vi "Dequeue if val.vi"(8 "error in (no error)":errorcluster, 11 "Queue in":refnum<queue>) -> (0 "error out":errorcluster, 3 "Queue out":refnum<queue>, 4 "Marin Serial Response":string)   [LabVIEW 2020]
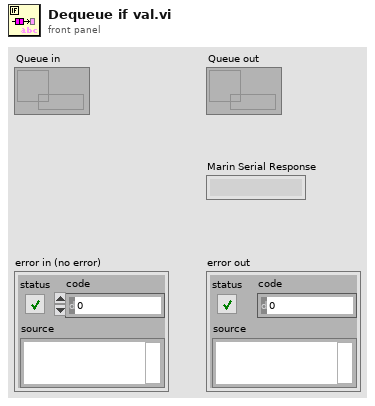
[diagram p1: front panel]
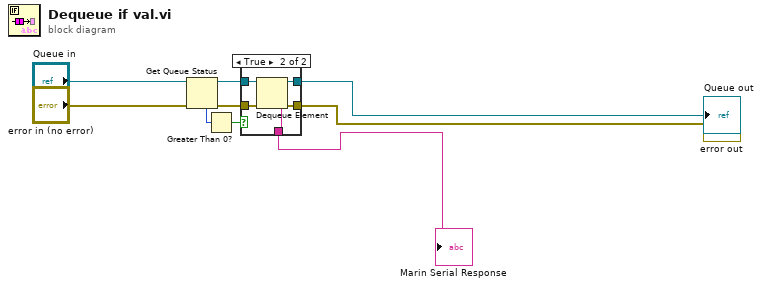
[diagram p0: block diagram]
diagram:
  n1 = Get Queue Status(queue="Queue in", error in (no error)="error in (no error)") -> (queue out=w5:refnum<queue>, error out=w4:errorcluster, # elements in queue=w8:i32)  [unwired: 1 in, 5 out]
  n2 = Greater Than 0?(x=w8) -> (x > 0?=w9:bool)
  n3 = case shown="True" w9 {
    tunnel: [w10 w16] -> w1
    tunnel: [w11 w15] -> w2
    tunnel: [_ w14] -> w3
    tunnel: w4 -> [w10 w13]
    tunnel: w5 -> [w11 w12]
    frame False {
    }
    frame True {
      n4 = Dequeue Element(queue=w12, error in (no error)=w13) -> (queue out=w15:refnum<queue>, element=w14:string, error out=w16:errorcluster)  [unwired: 1 in, 1 out]
    }
  }
  "Marin Serial Response" <- w3
  "Queue out" <- w2
  "error out" <- w1
